vi "EXDIR-YAML_LinesToArray.vi"(11 "array of lines in":string[](array[string])) -> (2 "ARRAY OF CLUSTERS":T1(array[cluster]), 3 "Array":variant[](array[variant]))   [LabVIEW 2016]
panel:
  out "ARRAY ELEMENTS":string[][](array[string])
  out "dashes line indices":i32[](array[numeric])
  out "test array out":string[](array[string])
  in  "spreadsheet string":string
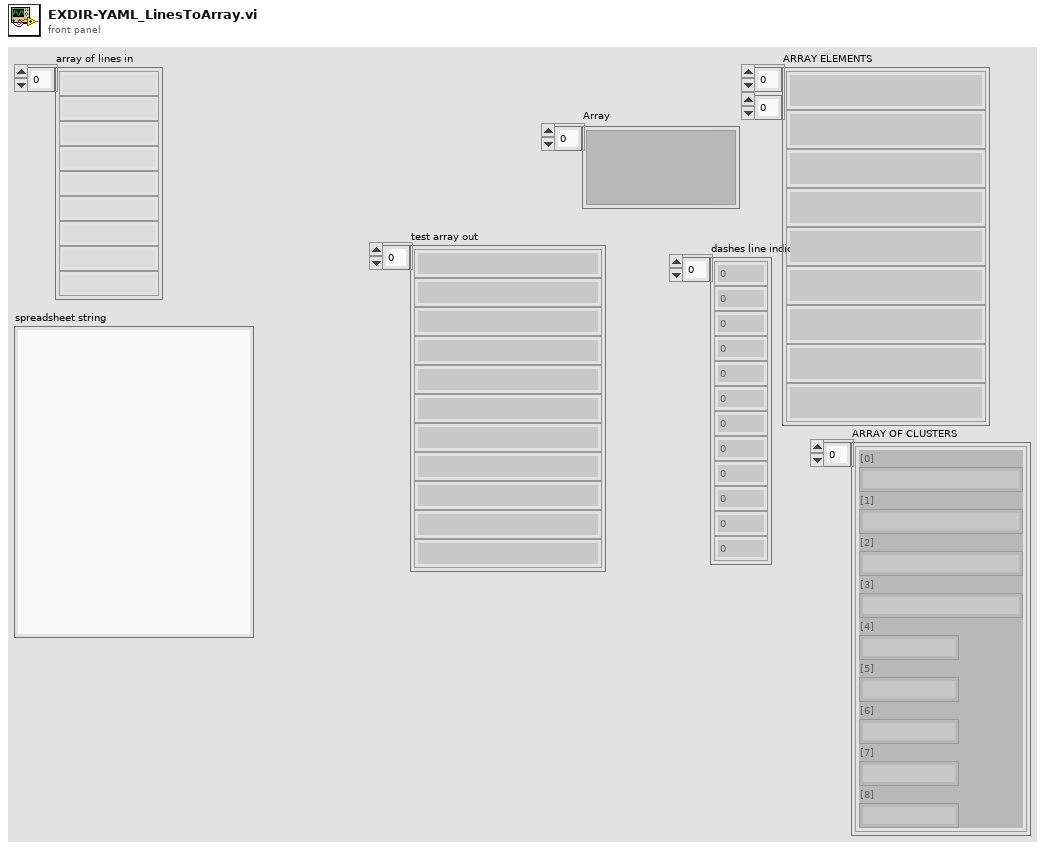
[diagram p1: front panel]
types:
  T1 = cluster{"[0]":string, "[1]":string, "[2]":string, "[3]":string, "[4]":string, "[5]":string, "[6]":string, "[7]":string, "[8]":string}[]
  T2 = cluster{"[0]":string, "[1]":string, "[2]":string, "[3]":string, "[4]":string, "[5]":string, "[6]":string, "[7]":string, "[8]":string}
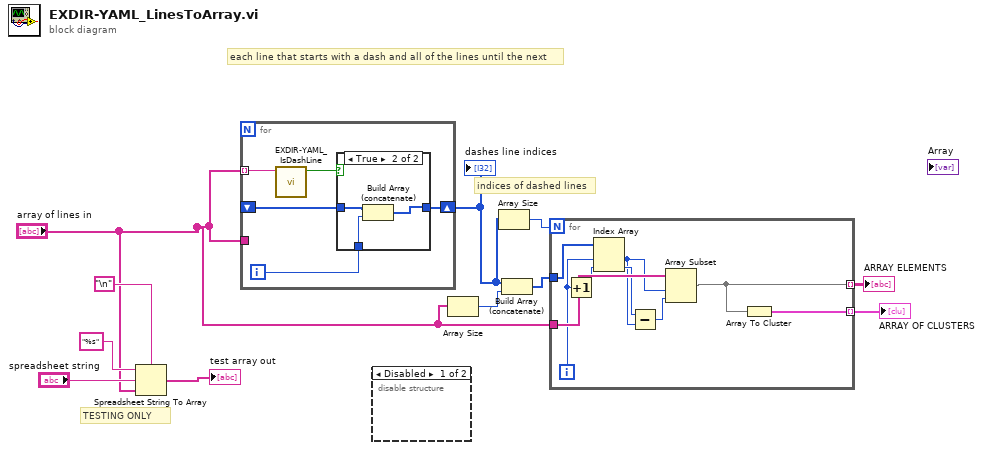
[diagram p0: block diagram]
diagram:
  # "TESTING ONLY"
  # "indices of dashed lines"
  # "each line that starts with a dash and all of the lines until the next"
  n1 = Spreadsheet String To Array(delimiter (Tab)="\n", format string="%s", spreadsheet string="spreadsheet string", array type (2D Dbl)="array of lines in") -> (array=→"test array out":string[])
  n2 = for {
    tunnel: "array of lines in" -> [w16] mode=indexing
    tunnel: "array of lines in" -> [_]
    shift-right: [w13] -> w6
    shift-left: _ -> [w14]
    i -> [w12]
    n3 = call "EXDIR-YAML_IsDashLine.vi"("Line"=w16) -> ("line starts with dash"=w15:bool)  [unwired: 10 in]
    n4 = case shown="True" w15 {
      tunnel: w14 -> [w17 w20]
      tunnel: [w17 w19] -> w13
      tunnel: w12 -> [_ w18]
      frame False {
      }
      frame True {
        n5 = Build Array (concatenate)(w20, w18) -> (w19:i32[])
      }
    }
  }
  "dashes line indices" <- w6
  n6 = disable-structure shown="Disabled" {
    frame Disabled {
    }
    frame Enabled {
    }
  }
  n7 = Array Size(array="array of lines in") -> (size(s)=w7:i32)
  n8 = Array Size(array=w6) -> (size(s)=w5:i32)
  n9 = Build Array (concatenate)(w6, w7) -> (w8:i32[])
  n10 = for {
    N: w5 -> [_]
    tunnel: w8 -> [w28]
    tunnel: "array of lines in" -> [w29]
    tunnel: [w22] -> w4 mode=indexing
    tunnel: [w21] -> w3 mode=indexing
    i -> [w26]
    n11 = Increment(x=w26) -> (x+1=w27:i32)
    n12 = Index Array(array=w28, index #1=w26, index #2=w27) -> (element #1=w24:i32, element #2=w25:i32)
    n13 = Subtract(x=w25, y=w24) -> (x-y=w23:i32)
    n14 = Array Subset(array=w29, index=w24, length=w23) -> (w22:string[])
    n15 = Array To Cluster(array=w22) -> (cluster=w21:T2)
  }
  "ARRAY ELEMENTS" <- w4
  "ARRAY OF CLUSTERS" <- w3
